vi "strToArrayValue.vi"(11 "String":string) -> (3 "Array":dbl[](array[numeric]))   [LabVIEW 2016]
doc: "Get the string data as the array."
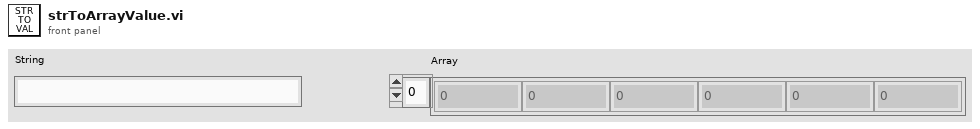
[diagram p1: front panel]
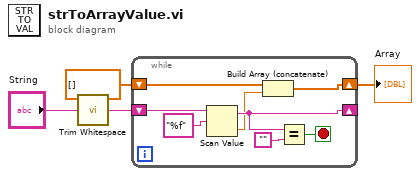
[diagram p0: block diagram]
diagram:
  n1 = call <vilib>:"Trim Whitespace.vi"("string"="String") -> ("trimmed string"=w4:string)  [unwired: 1 in]
  n2 = while {
    shift-right: [w10] -> _
    shift-left: w4 -> [w12]
    shift-right: [w5] -> w1
    shift-left: dbl[] [] -> [w7]
    stop <- w8 stop-if-true
    n3 = Scan Value(string=w12, format string="%f") -> (output string=w10:string, value=w6:dbl)  [unwired: 1 in]
    n4 = Build Array (concatenate)(w7, w6) -> (w5:dbl[])
    n5 = Equal?(x=w10, y="") -> (x = y?=w8:bool)
  }
  "Array" <- w1
